vi "Wait till chilled water below.vi"(3 "Mode":T5, 5 "Traverse line In":T2 {"Carrier_2 Q (l/min)" format="%#.2f"; "Row Duration (mins)" format="%#.1f"; "Row No" min=0; "Trace Gas Concentration (%)" min=0.0 format="%#_4f"; "Carrier_1 Q (l/min)" format="%#.2f"; "Tunnel Speed" format="%#.2f"; "Start X" format="%#.2f"; "Start Y" format="%#.2f"; "Start Z" format="%#.2f"; "End X" format="%#.2f"; "End Y" format="%#.2f"; "End Z" format="%#.2f"; "Averaging time (min)" min=0.0 format="%#.2f"}) -> (0 "Error Message":string, 1 "Status":T1, 2 "Traverse line Out":T2 {"Carrier_2 Q (l/min)" format="%#.2f"; "Row Duration (mins)" format="%#.1f"; "Row No" min=0; "Trace Gas Concentration (%)" min=0.0 format="%#_4f"; "Carrier_1 Q (l/min)" format="%#.2f"; "Tunnel Speed" format="%#.2f"; "Start X" format="%#.2f"; "Start Y" format="%#.2f"; "Start Z" format="%#.2f"; "End X" format="%#.2f"; "End Y" format="%#.2f"; "End Z" format="%#.2f"; "Averaging time (min)" min=0.0 format="%#.2f"})   [LabVIEW 2017]
uses:
  Gen Trav/Traverse_cluster.ctl
  Gen Trav/Spacing.ctl
  Controls/Multi_run_mode.ctl
  Controls/User_Specific_mode.ctl
  Gen Trav/Multi_Run_Status.ctl
  ADAM Client/Sub VIs/ADAM Controls/Tunnel_speed_mode.ctl
panel:
  out "Initial Hydrosonic setting":dbl
  in  "stop":bool
  out "Chilled water temp":dbl(graph)
  out "Initial Uni Chilled water temp":dbl
  out "Initial Tunnel Speed":dbl
  # "X           Y            Z"
  # "Start"
  # "End"
  # "X           Y            Z"
  # "Start"
  # "End"
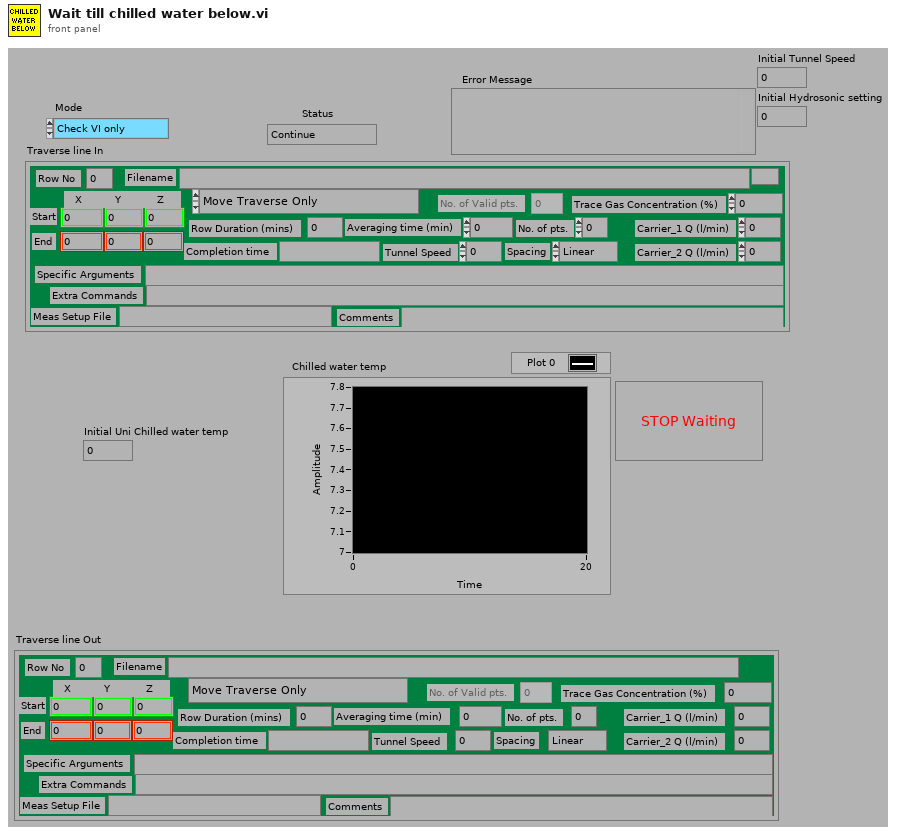
[diagram p1: front panel]
types:
  T1 = typedef "Multi_Run_Status.ctl" = enum16{"Continue", "Continue with Error", "Jump to Next Point", "Jump to Next Row", "Jump To Fall Back", "Terminate Run"}
  T2 = typedef "Traverse_cluster.ctl" = cluster{"Start X":sgl, "Start Y":sgl, "Start Z":sgl, "End X":sgl, "End Y":sgl, "End Z":sgl, "No. of pts.":i32, "Spacing":T3, "Filename":path, "Tunnel Speed":dbl, "Averaging time (min)":dbl, "Extra Commands":string, "Carrier_1 Q (l/min)":dbl, "Carrier_2 Q (l/min)":dbl, "Trace Gas Concentration (%)":dbl, "Specific Arguments":string, "Comments":string, "Row No":i32, "Row Type Selector":T4, "Completion time":string, "Row Duration (mins)":dbl, "No. of Valid pts.":i32, "Meas Setup File":string}
  T3 = typedef "Spacing.ctl" = enum16{"Linear", "Log", "Gauss", "Specified", "N/A"}
  T4 = typedef "Multi_run_mode.ctl" = enum16{"Move Traverse Only", "Set Tunnel Speed Only", "Set Source Only", "Set Measurement Conditions", "Single Measurement", "Vertical Profile", "Lateral Profile", "Longitudinal Profile", "Explore Volume", "Multi-Axis Profile", "Auto Calibrate", "Meas Fast FID Bkgnd", "Check Beam Power", "Scanning Valve Measurement", "Run VI Named:", "Set ADAM Ch", "Wait (minutes)", "Send Message", "Synchronize With:", "Fall Back to this Row", "Turn Off Row Repeating", "Blank Row", "Traverse 3D Volume"}
  T5 = typedef "User_Specific_mode.ctl" = enum16{"Check VI only", "Run VI"}
  T6 = typedef "Tunnel_speed_mode.ctl" = enum16{"Set Speed", "Set Speed then wait", "Is tunnel speed allowable?"}
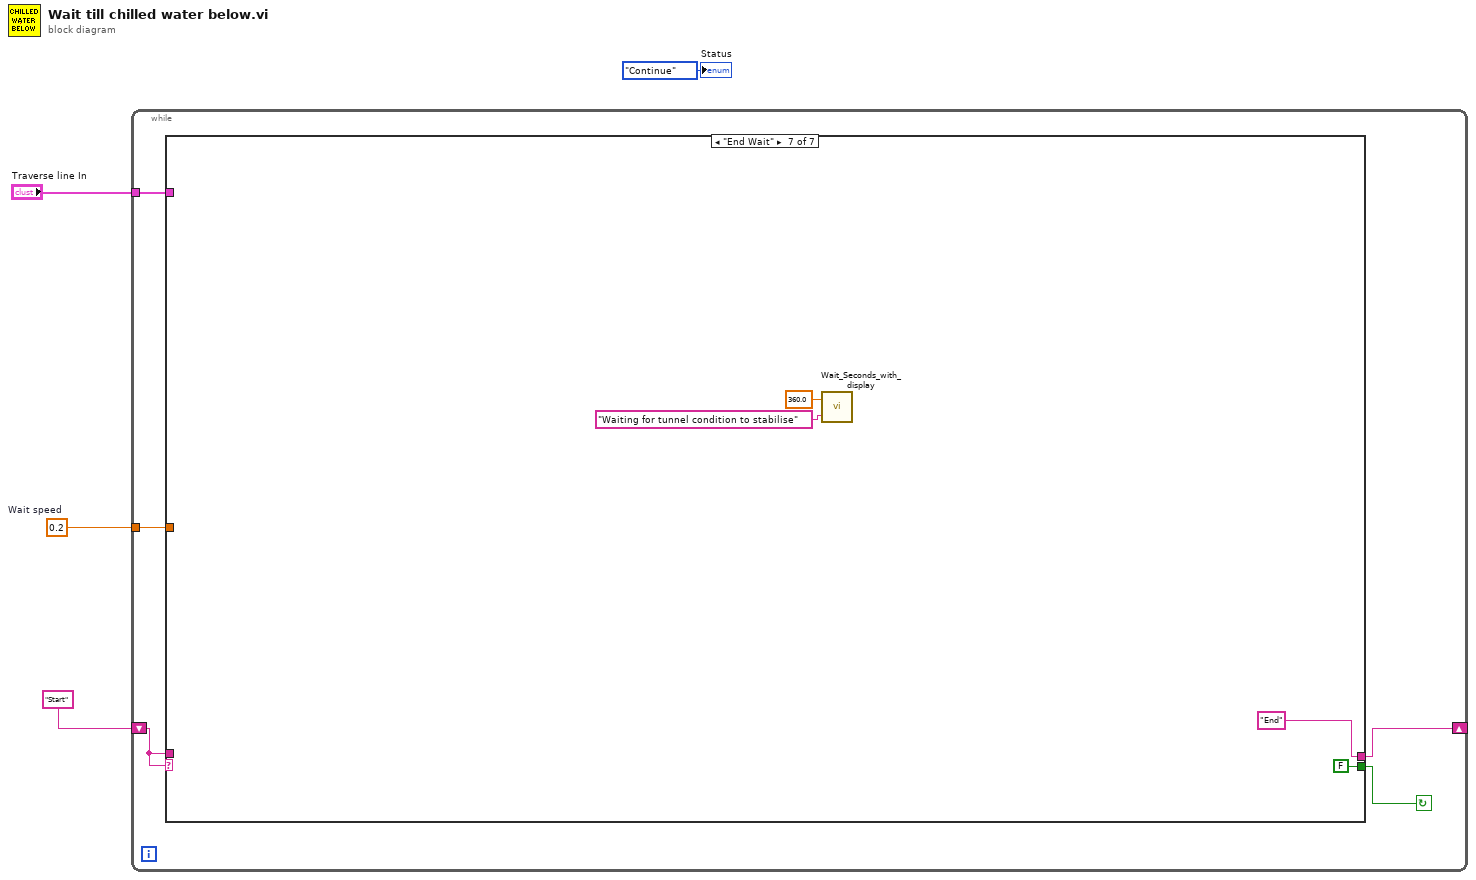
[diagram p0: block diagram]
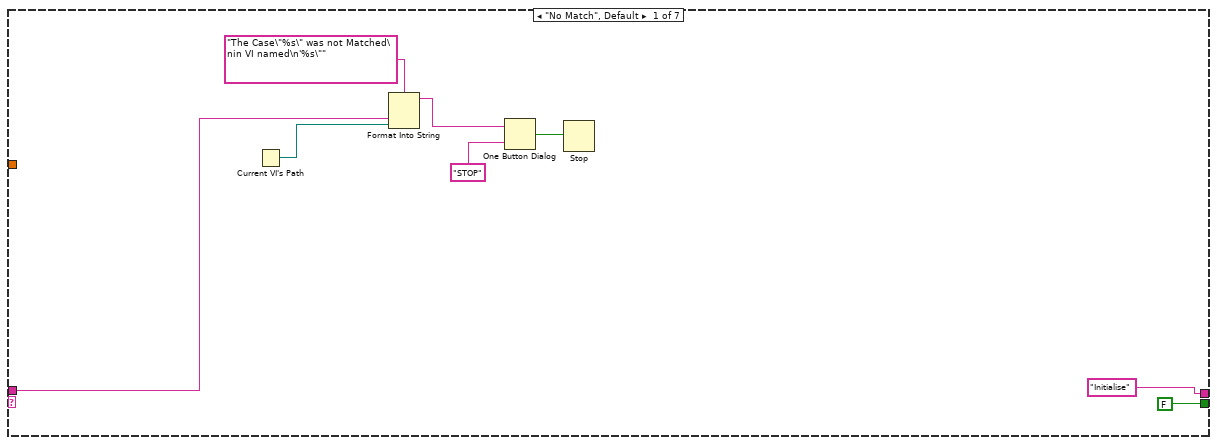
[diagram p2: hidden frame]
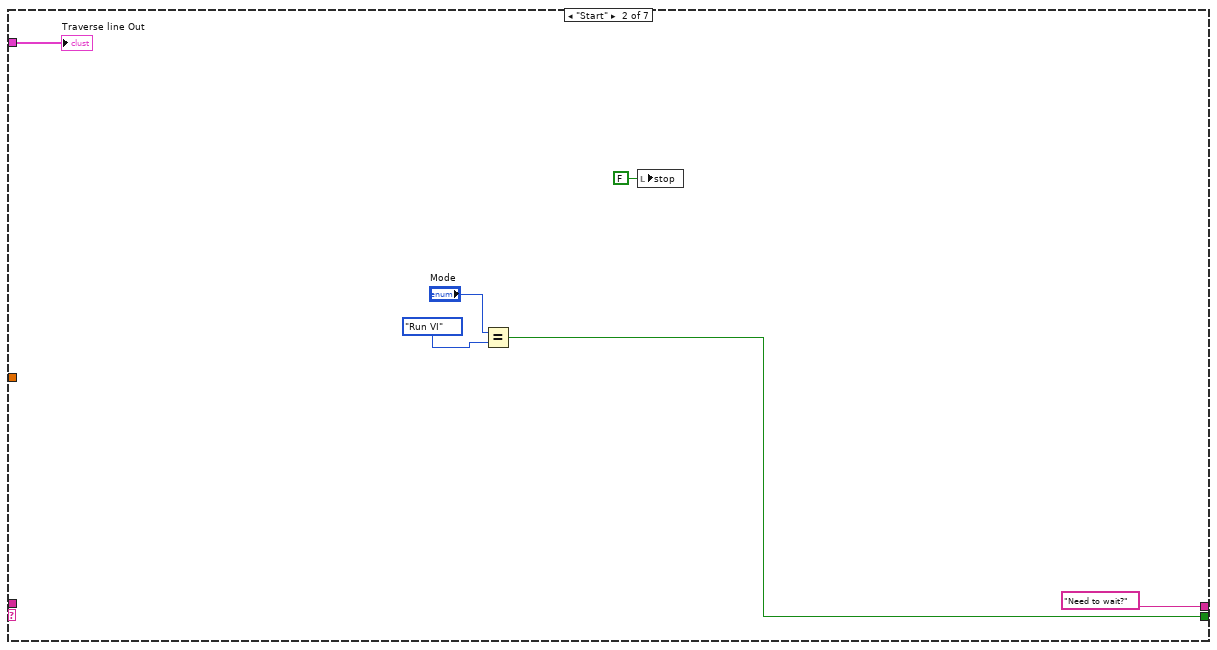
[diagram p3: hidden frame]
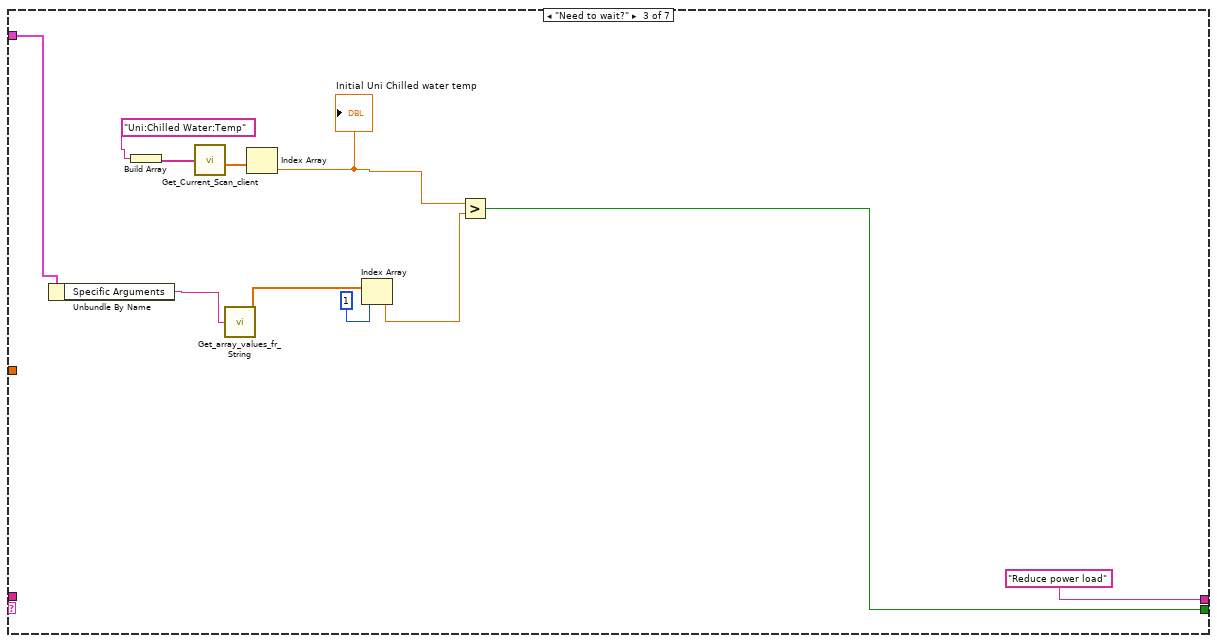
[diagram p4: hidden frame]
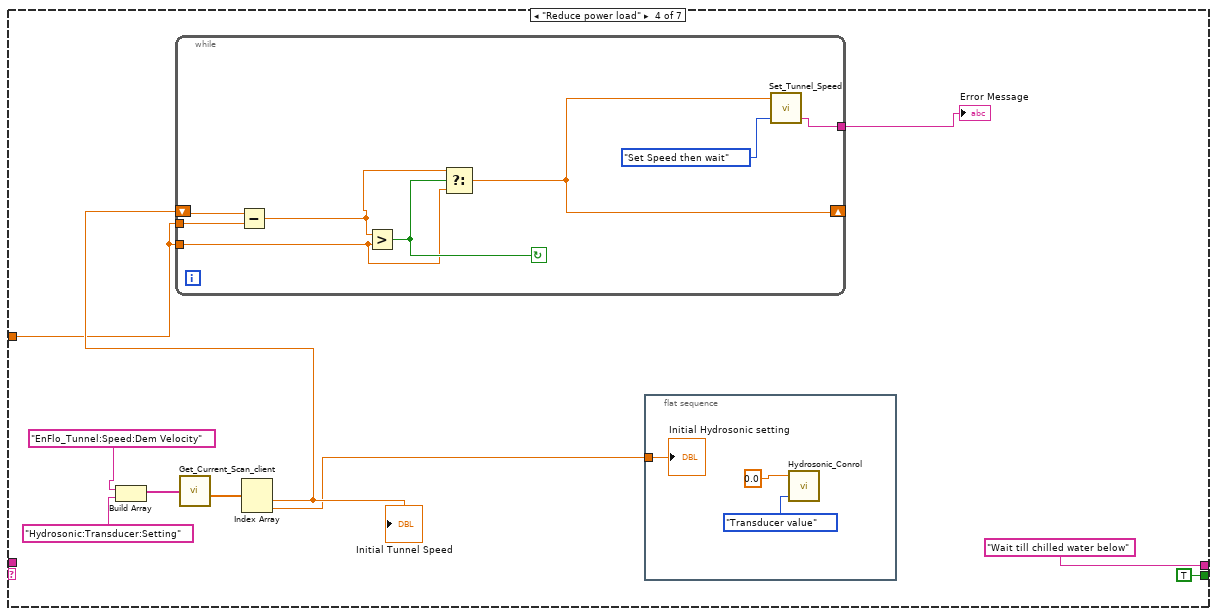
[diagram p5: hidden frame]
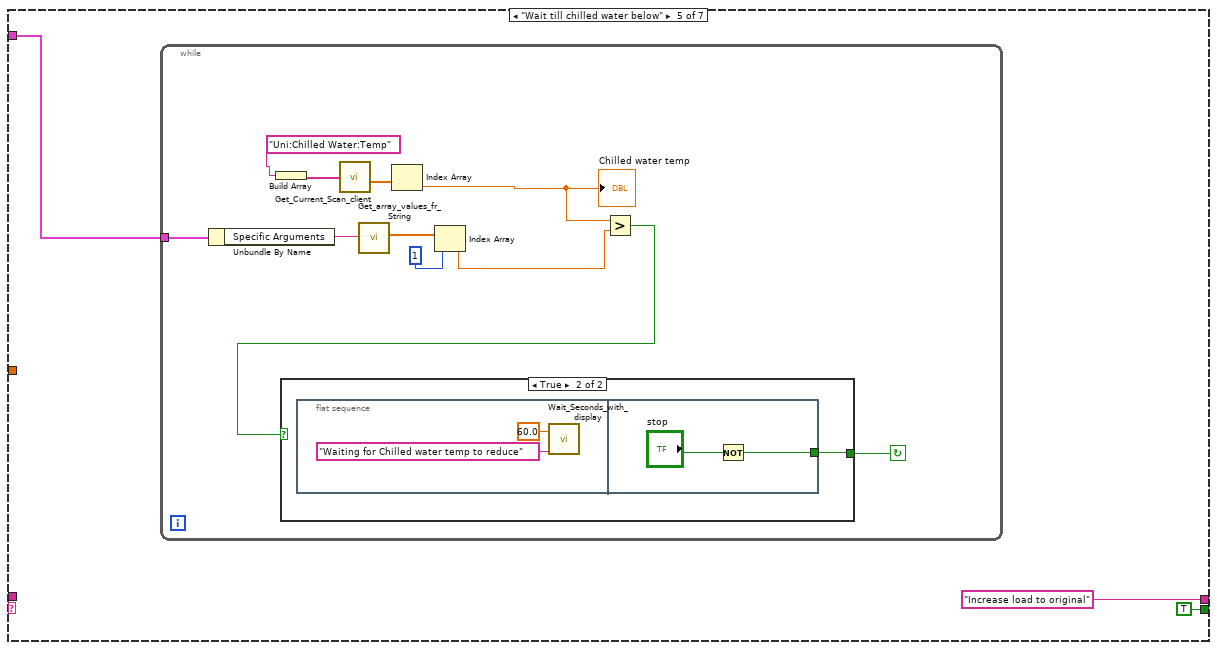
[diagram p6: hidden frame]
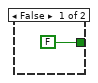
[diagram p7: hidden frame]
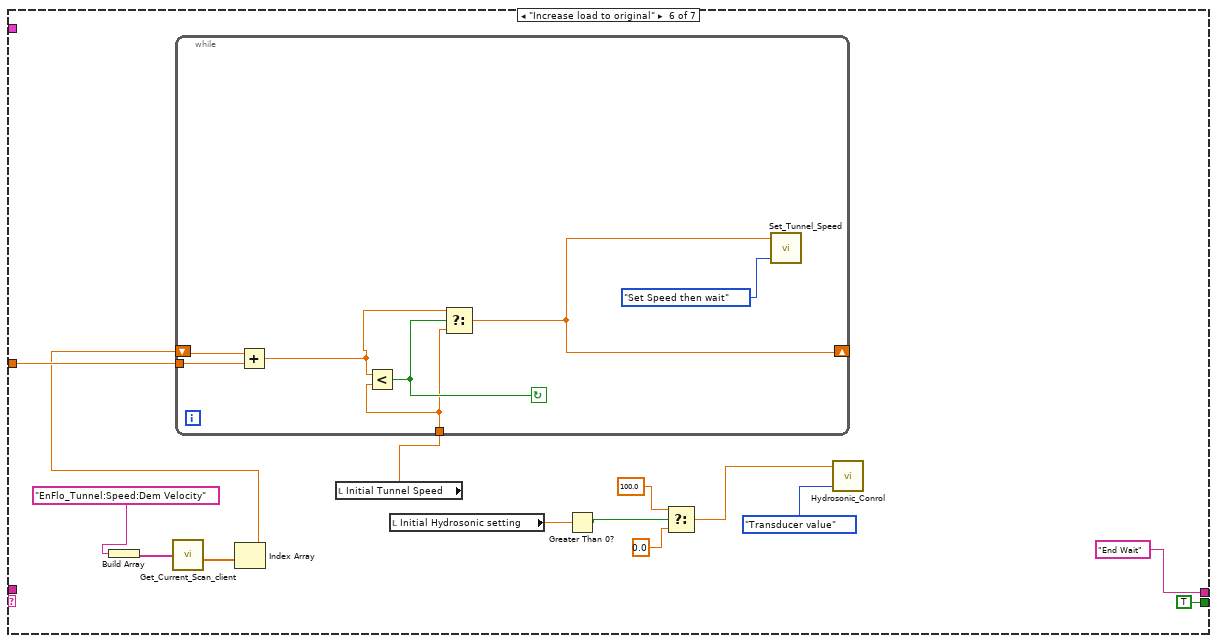
[diagram p8: hidden frame]
diagram:
  w2 = 0.2  # Wait speed
  n1 = while {
    shift-left: "Start" -> [w7]
    shift-right: [w8] -> _
    tunnel: "Traverse line In" -> [w6]
    tunnel: w2 -> [w5]
    stop <- w9 continue-if-true
    n2 = case shown="\"End Wait\"" w7 {
      tunnel: [FALSE w20 w25 TRUE TRUE TRUE FALSE] -> w9
      tunnel: ["Initialise" "Need to wait?" "Reduce power load" "Wait till chilled water below" "Increase load to original" "End Wait" "End"] -> w8
      tunnel: w7 -> [w12 _ _ _ _ _ _]
      tunnel: w6 -> [_ w19 w24 _ w57 _ _]
      tunnel: w5 -> [_ _ _ w39 _ w86 _]
      frame "No Match", Default {
        n3 = Current VI's Path() -> (path=w11:path)
        n4 = Format Into String(format string="The Case\"%s\" was not Matched\nin VI named\n'%s\"" ("Format String"), w12, w11) -> (resulting string=w15:string)  [unwired: 2 in, 1 out]
        n5 = One Button Dialog(message=w15, button name ("OK")="STOP") -> (true=w13:bool)
        n6 = Stop(stop? (T)=w13) -> ()
      }
      frame "Start" {
        n7 = Equal?(x="Mode", y=User_Specific_mode."Run VI" ("Mode")) -> (x = y?=w20:bool)
        n8 = local write "stop"(FALSE ("stop")) -> ()
        "Traverse line Out" <- w19
      }
      frame "Need to wait?" {
        n9 = Unbundle By Name(w24) -> ("Specific Arguments"=w29:string)
        n10 = Build Array("Uni:Chilled Water:Temp") -> (w30:string[])
        n11 = call "Get_Current_Scan_client.vi"("ADAM Ch Names"=w30) -> ("Numerical Values"=w31:dbl[])  [unwired: 1 in, 2 out]
        n12 = call "Get_array_values_fr_String.vi"("String Value"=w29) -> ("Numeric Array"=w27:dbl[])  [unwired: 1 out]
        n13 = Index Array(array=w31) -> (element=w33:dbl)  [unwired: 1 in]
        "Initial Uni Chilled water temp" <- w33
        n14 = Index Array(array=w27, index=1) -> (element=w26:dbl)
        n15 = Greater?(x=w33, y=w26) -> (0:w25:bool)
      }
      frame "Reduce power load" {
        n16 = Build Array("EnFlo_Tunnel:Speed:Dem Velocity", "Hydrosonic:Transducer:Setting") -> (w41:string[])
        n17 = call "Get_Current_Scan_client.vi"("ADAM Ch Names"=w41) -> ("Numerical Values"=w42:dbl[])  [unwired: 1 in, 2 out]
        n18 = Index Array(array=w42) -> (element #1=w40:dbl, element #2=w35:dbl)  [unwired: 2 in]
        "Initial Tunnel Speed" <- w40
        n19 = while {
          shift-right: [w51] -> _
          shift-left: w40 -> [w55]
          tunnel: w39 -> [w50]
          tunnel: w39 -> [w49]
          tunnel: [w48] -> w37
          stop <- w52 continue-if-true
          n20 = Subtract(x=w55, y=w50) -> (x-y=w53:dbl)
          n21 = Greater?(x=w53, y=w49) -> (0:w52:bool)
          n22 = Select(t=w53, s=w52, f=w49) -> (s? t:f=w51:dbl)
          n23 = call "Set_Tunnel_Speed.vi"("Mode"=Tunnel_speed_mode."Set Speed then wait" ("Mode 2"), "Tunnel Velocity m/s"=w51) -> ("Error String"=w48:string)  [unwired: 2 in, 1 out]
        }
        "Error Message" <- w37
        n24 = flat-sequence {
          tunnel: w35 -> [w45]
          frame #0 {
            n25 = call "Hydrosonic_Conrol.vi"("Input Mode"=enum16{"Desired Frequency", "Transducer value"}."Transducer value", "Desired Value"=0.0 ("Set output")) -> ()  [unwired: 2 in, 2 out]
            "Initial Hydrosonic setting" <- w45
          }
        }
      }
      frame "Wait till chilled water below" {
        n26 = while {
          tunnel: w57 -> [w62]
          stop <- w59 continue-if-true
          n27 = Unbundle By Name(w62) -> ("Specific Arguments"=w66:string)
          n28 = Build Array("Uni:Chilled Water:Temp") -> (w67:string[])
          n29 = call "Get_Current_Scan_client.vi"("ADAM Ch Names"=w67) -> ("Numerical Values"=w68:dbl[])  [unwired: 1 in, 2 out]
          n30 = call "Get_array_values_fr_String.vi"("String Value"=w66) -> ("Numeric Array"=w64:dbl[])  [unwired: 1 out]
          n31 = Index Array(array=w68) -> (element=w61:dbl)  [unwired: 1 in]
          "Chilled water temp" <- w61
          n32 = Index Array(array=w64, index=1) -> (element=w63:dbl)
          n33 = Greater?(x=w61, y=w63) -> (0:w60:bool)
          n34 = case shown="True" w60 {
            tunnel: [FALSE w71] -> w59
            frame False {
            }
            frame True {
              n35 = flat-sequence {
                tunnel: [w74] -> w71
                frame #0 {
                  n36 = call "Wait_Seconds_with_display.vi"("Message"="Waiting for Chilled water temp to reduce", "Seconds to wait"=60.0) -> ()  [unwired: 1 in, 1 out]
                }
                frame #1 {
                  n37 = Not(x="stop") -> (.not. x?=w74:bool)
                }
              }
            }
          }
        }
      }
      frame "Increase load to original" {
        n38 = Build Array("EnFlo_Tunnel:Speed:Dem Velocity") -> (w87:string[])
        n39 = call "Get_Current_Scan_client.vi"("ADAM Ch Names"=w87) -> ("Numerical Values"=w88:dbl[])  [unwired: 1 in, 2 out]
        n40 = Index Array(array=w88) -> (element=w85:dbl)  [unwired: 1 in]
        n41 = local read "Initial Tunnel Speed"() -> (w77:dbl)
        n42 = while {
          shift-right: [w92] -> _
          shift-left: w85 -> [w96]
          tunnel: w86 -> [w91]
          tunnel: w77 -> [w90]
          stop <- w93 continue-if-true
          n43 = Add(x=w96, y=w91) -> (x+y=w94:dbl)
          n44 = Less?(x=w94, y=w90) -> (x < y?=w93:bool)
          n45 = Select(t=w94, s=w93, f=w90) -> (s? t:f=w92:dbl)
          n46 = call "Set_Tunnel_Speed.vi"("Mode"=Tunnel_speed_mode."Set Speed then wait" ("Mode 2"), "Tunnel Velocity m/s"=w92) -> ()  [unwired: 2 in, 2 out]
        }
        n47 = local read "Initial Hydrosonic setting"() -> (w76:dbl)
        n48 = Greater Than 0?(x=w76) -> (x > 0?=w78:bool)
        n49 = Select(t=100.0 ("Set output"), s=w78, f=0.0 ("Set output")) -> (s? t:f=w79:dbl)
        n50 = call "Hydrosonic_Conrol.vi"("Input Mode"=enum16{"Desired Frequency", "Transducer value"}."Transducer value", "Desired Value"=w79) -> ()  [unwired: 2 in, 2 out]
      }
      frame "End Wait" {
        n51 = call "Wait_Seconds_with_display.vi"("Message"="Waiting for tunnel condition to stabilise", "Seconds to wait"=360.0) -> ()  [unwired: 1 in, 1 out]
      }
    }
  }
  "Status" <- Multi_Run_Status."Continue" ("Status")
